vi "Simple Setpoint Omega Controller.vi"(9 "Set Point Temperature":dbl=25.0 min=0.0 max=100000.0 step=0.1 format="%.1f", 11 "VISA resource name":refnum<visa-resource-name>) -> ()   [LabVIEW 2011]
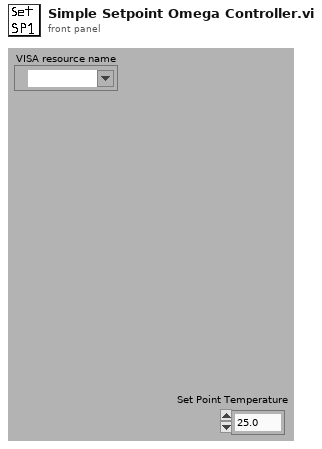
[diagram p1: front panel]
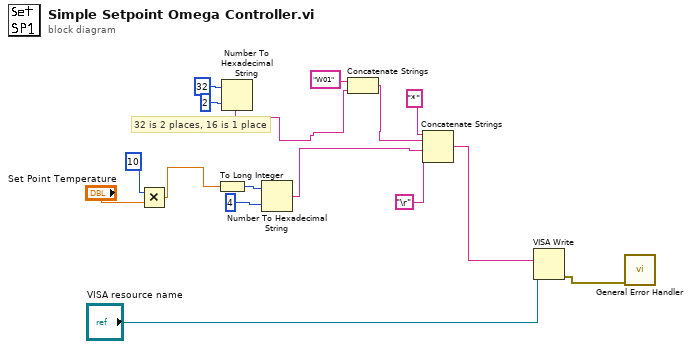
[diagram p0: block diagram]
diagram:
  # "32 is 2 places, 16 is 1 place"
  n1 = Multiply(x=i16 10, y="Set Point Temperature") -> (x*y=w5:dbl)
  n2 = To Long Integer(number=w5) -> (32bit integer=w6:i32)
  n3 = Number To Hexadecimal String(1:i16 2 ("width (-)"), 2:32 ("number")) -> (0:w10:string)
  n4 = Number To Hexadecimal String(1:i16 4 ("width (-)"), 2:w6) -> (0:w4:string)
  n5 = Concatenate Strings("W01" ("Substring"), w10) -> (w13:string)
  n6 = Concatenate Strings("*", w13, w4, "\r") -> (w2:string)
  n7 = VISA Write(VISA resource name="VISA resource name", write buffer=w2) -> (error out=w1:errorcluster)  [unwired: 1 in, 2 out]
  n8 = call <vilib>:"General Error Handler.vi"("error in (no error)"=w1) -> ()  [unwired: 1 in, 14 out]
